vi "Get Measurement Details.vi"(8 "error in":errorcluster) -> (0 "error out":errorcluster, 3 "measurement_details":T1)   [LabVIEW 2020, in "Line Regulation.lvlib"]
uses:
  Line Regulation.lvlib
  RPC Messages/ni_measurements_v1_MeasurementDetails.ctl
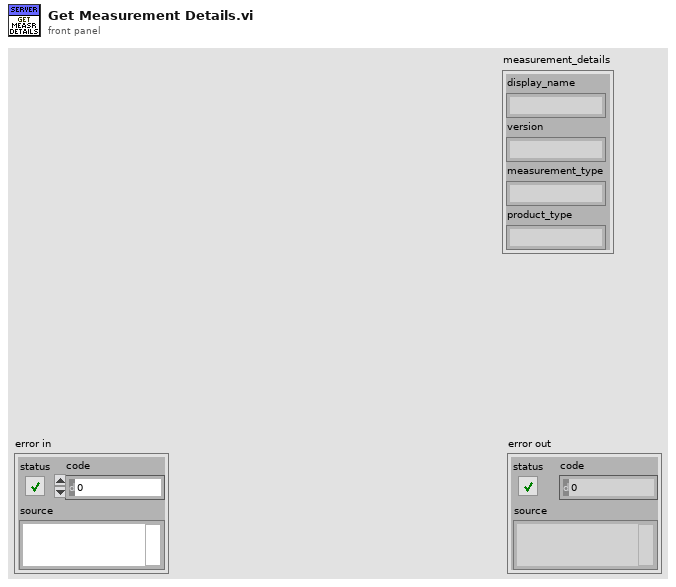
[diagram p1: front panel]
types:
  T1 = typedef "Line Regulation.lvlib/ni_measurements_v1_MeasurementDetails.ctl" = cluster{"display_name":string, "version":string, "measurement_type":string, "product_type":string}
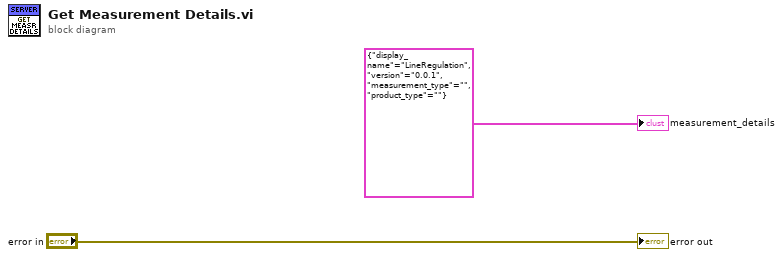
[diagram p0: block diagram]
diagram:
  "error out" <- "error in"
  "measurement_details" <- T1 {"display_name"="LineRegulation", "version"="0.0.1", "measurement_type"="", "product_type"=""} ("ni_measurements_v1_MeasurementDetails")
